vi "Gradient-Ascent_alignment-max.vi"() -> (2 "x":dbl, 3 "y":dbl)   [LabVIEW 2024]
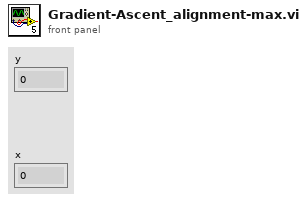
[diagram p1: front panel]
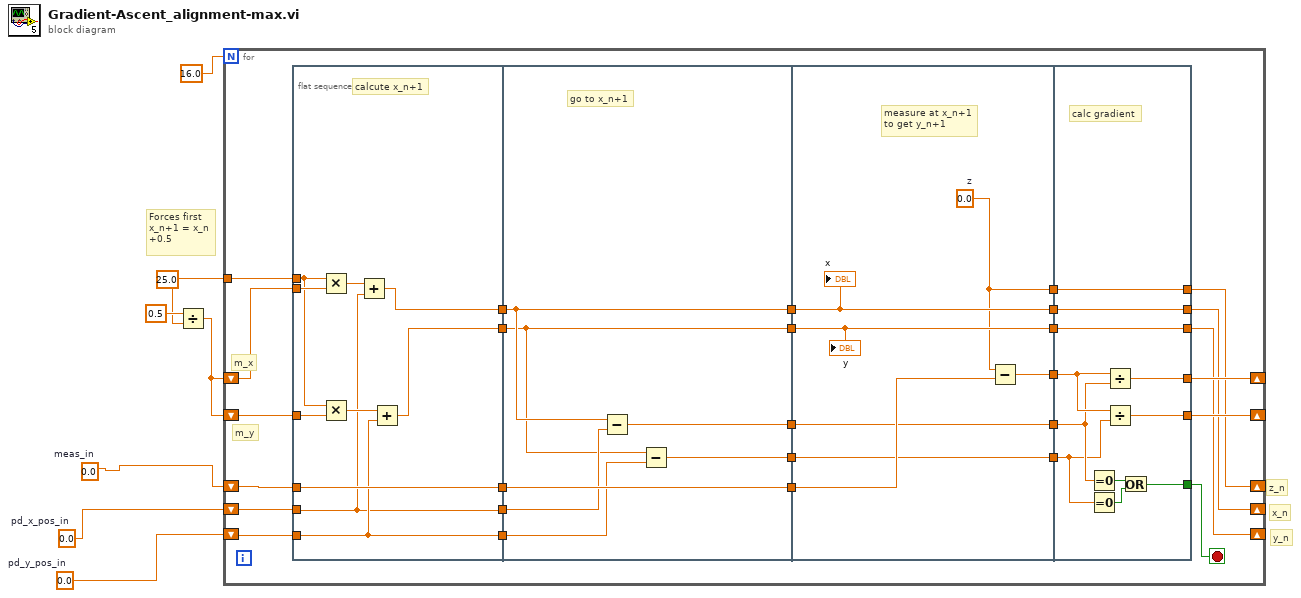
[diagram p0: block diagram]
diagram:
  w3 = 25.0 ("k 2")
  w7 = 0.0  # meas_in
  w6 = 0.0  # pd_y_pos_in
  w5 = 0.0  # pd_x_pos_in
  # "y_n"
  # "x_n"
  # "z_n"
  # "Forces first x_n+1 = x_n +0.5"
  n1 = Divide(x=0.5, y=w3) -> (x/y=w1:dbl)
  n2 = for {
    N: 16.0 ("N trials 2") -> [_]
    shift-right: [w18] -> _
    shift-left: w5 -> [w30]
    shift-right: [w19] -> _
    shift-left: w7 -> [w31]
    tunnel: w3 -> [w35]
    shift-right: [w17] -> _
    shift-left: w6 -> [w27]
    shift-right: [w22] -> _
    shift-left: w1 -> [w20]
    shift-right: [w23] -> _
    shift-left: w1 -> [w21]
    stop <- w13 stop-if-true
    # "m_y"
    # "m_x"
    n3 = flat-sequence {
      tunnel: w35 -> [w40]
      tunnel: [w45] -> w34
      tunnel: w31 -> [w44]
      tunnel: [w44] -> w32
      tunnel: w30 -> [w36]
      tunnel: [w36] -> w29
      tunnel: [w38] -> w28
      tunnel: w27 -> [w38]
      tunnel: [w43] -> w26
      tunnel: w21 -> [w42]
      tunnel: w20 -> [w41]
      tunnel: [w47] -> w16
      tunnel: [w52] -> w15
      tunnel: [w46] -> w14
      tunnel: [w51] -> w11
      tunnel: [w50] -> w8
      tunnel: w26 -> [w46]
      tunnel: w28 -> [w48]
      tunnel: w29 -> [w49]
      tunnel: w32 -> [w52]
      tunnel: w34 -> [w47]
      tunnel: w16 -> [w59]
      tunnel: [w59] -> w33
      tunnel: w15 -> [w57]
      tunnel: w14 -> [w58]
      tunnel: [w58] -> w25
      tunnel: [w53] -> w24
      tunnel: [w56] -> w12
      tunnel: w11 -> [w55]
      tunnel: [w55] -> w10
      tunnel: [w54] -> w9
      tunnel: w8 -> [w54]
      tunnel: w33 -> [w68]
      tunnel: [w68] -> w18
      tunnel: w25 -> [w67]
      tunnel: [w67] -> w17
      tunnel: w24 -> [w66]
      tunnel: [w66] -> w19
      tunnel: [w70] -> w23
      tunnel: [w69] -> w22
      tunnel: [w63] -> w13
      tunnel: w12 -> [w62]
      tunnel: w10 -> [w61]
      tunnel: w9 -> [w60]
      frame #0 {
        # "calcute x_n+1"
        n4 = Multiply(x=w40, y=w42) -> (x*y=w37:dbl)
        n5 = Multiply(x=w40, y=w41) -> (x*y=w39:dbl)
        n6 = Add(x=w37, y=w36) -> (x+y=w45:dbl)
        n7 = Add(x=w39, y=w38) -> (x+y=w43:dbl)
      }
      frame #1 {
        # "go to x_n+1"
        n8 = Subtract(x=w47, y=w49) -> (x-y=w51:dbl)
        n9 = Subtract(x=w46, y=w48) -> (x-y=w50:dbl)
      }
      frame #2 {
        w53 = 0.0  # z
        # "measure at x_n+1\nto get y_n+1"
        n10 = Subtract(x=w53, y=w57) -> (x-y=w56:dbl)
        "x" <- w59
        "y" <- w58
      }
      frame #3 {
        # "calc gradient"
        n11 = Equal To 0?(x=w61) -> (x = 0?=w65:bool)
        n12 = Equal To 0?(x=w60) -> (x = 0?=w64:bool)
        n13 = Divide(x=w62, y=w61) -> (x/y=w70:dbl)
        n14 = Divide(x=w62, y=w60) -> (x/y=w69:dbl)
        n15 = Or(x=w65, y=w64) -> (x .or. y?=w63:bool)
      }
    }
  }
